vi "CustomConstructService.vi"() -> (2 "MicronMessageUE":refnum<user-event>, 3 "MicronGRPC out":refnum<class "MicronGRPC.lvclass">)   [LabVIEW 2019, in "MicronGRPCGeneratedServer.lvlib"]
uses:
  MicronGRPCGeneratedServer.lvlib
  RPC Service/MicronGRPC/MicronGRPC.lvclass
  Base/Server/Message/MessageBase.lvclass
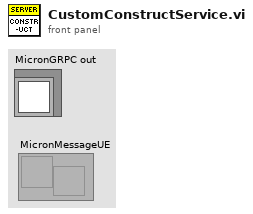
[diagram p1: front panel]
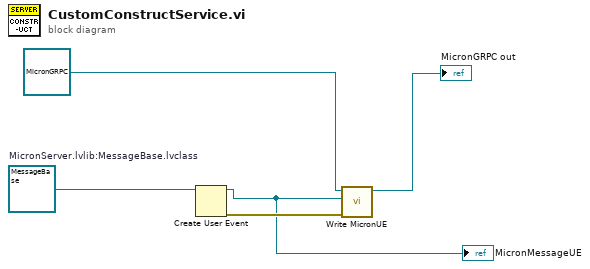
[diagram p0: block diagram]
diagram:
  w2 = refnum<class "MessageBase.lvclass"> refnum  # MicronServer.lvlib:MessageBase.lvclass
  n1 = Create User Event(user event datatype=w2) -> (user event=w1:refnum<user-event>, error out=w5:errorcluster)  [unwired: 1 in]
  "MicronMessageUE" <- w1
  n2 = call-dynamic "Write MicronUE.vi"("error in (no error)"=w5, "MicronUE"=w1, "MicronGRPC in"=refnum<class "MicronGRPC.lvclass"> refnum ("MicronGRPCGeneratedServer.lvlib:MicronGRPC.lvclass")) -> ("MicronGRPC out"=→"MicronGRPC out":refnum<class "MicronGRPC.lvclass">)  [unwired: 7 in, 1 out]
